vi "Initialize.vi"(8 "error in (no error)":errorcluster, 11 "Serial Config":T1={"Baud"=9600, "Flow Ctl"=0, "Parity"=0, "COM Port"="", "Address"=0} {"Parity" items=["None", "Odd", "Even"]; "Flow Ctl" items=["None"]; "Baud" items=["4800"=4800, "9600"=9600, "19200"=19200, "38400"=38400]}) -> (0 "error out":errorcluster, 3 "Serial Config 2":T1={"Baud"=9600, "Flow Ctl"=0, "Parity"=0, "COM Port"="", "Address"=0} {"Parity" items=["None", "Odd", "Even"]; "Flow Ctl" items=["None"]; "Baud" items=["4800"=4800, "9600"=9600, "19200"=19200, "38400"=38400]})   [LabVIEW 2014, in "Omega CN9600 series.lvclass"]
uses:
  Omega CN9600 series.lvclass
  Serial_Config_Omega.ctl
  <vilib>/Instr/_visa.llb/VISA Set IO Buffer Mask.ctl
  <vilib>/Utility/error.llb/Error Cluster From Error Code.vi
  <vilib>/ErrorRing/Error Ring.xnode
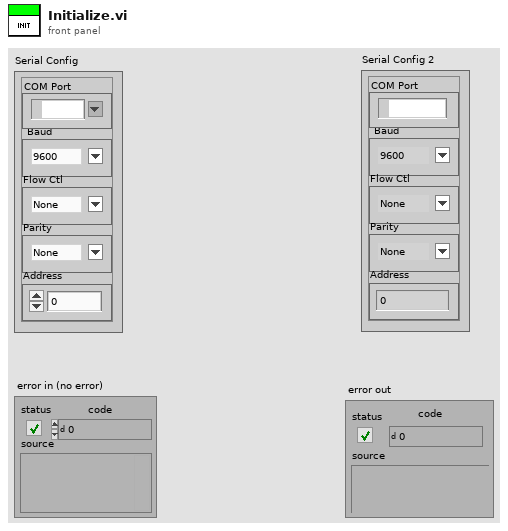
[diagram p1: front panel]
types:
  T1 = typedef "Omega CN9600 series.lvclass/Serial_Config_Omega.ctl" = cluster{"Baud":u32, "Flow Ctl":u16, "Parity":u16, "COM Port":refnum<visa-resource-name>, "Address":u8}
  T2 = typedef "VISA Set IO Buffer Mask.ctl" = u16
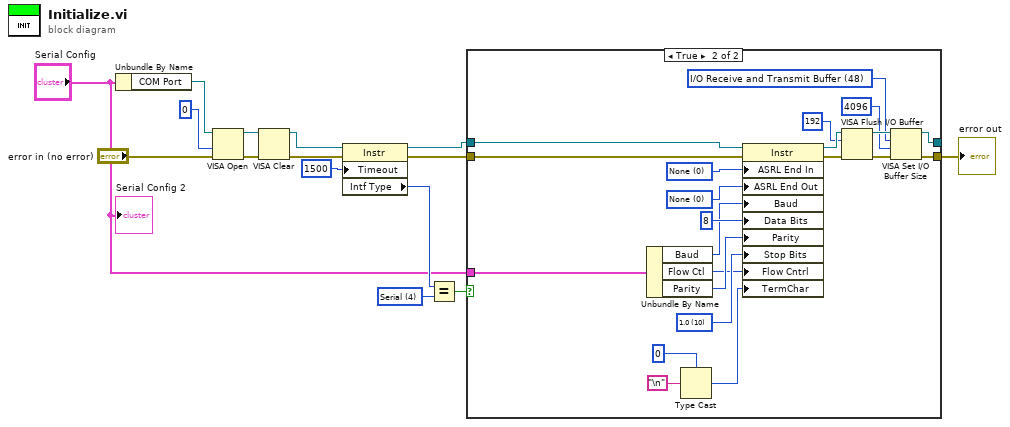
[diagram p0: block diagram]
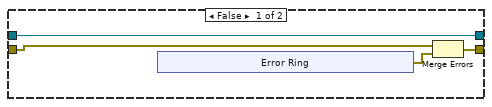
[diagram p2: hidden frame]
diagram:
  w7 = u16 4 items=["GPIB"=1, "VXI"=2, "GPIB-VXI"=3, "Serial"=4, "PXI"=5, "TCPIP"=6, "USB"=7] ("Interface Information:Interface Type")
  n1 = Unbundle By Name("Serial Config") -> ("COM Port"=w3:refnum<visa-resource-name>)
  n2 = VISA Open(access mode=0, error in (no error)="error in (no error)", VISA resource name=w3) -> (VISA resource name=w12:refnum<visa-resource-name>, error out=w13:errorcluster)  [unwired: 2 in]
  n3 = VISA Clear(VISA resource name=w12, error in (no error)=w13) -> (VISA resource name out=w11:refnum<visa-resource-name>, error out=w10:errorcluster)
  n4 = property class="Instr"(reference=w11, error in=w10, "Timeout"=u32 1500 ("General Settings:Timeout Value")) -> (reference out=w5:refnum<visa-resource-name>, error out=w4:errorcluster, "Intf Type"=w8:u16)
  n5 = Equal?(x=w8, y=w7) -> (x = y?=w6:bool)
  n6 = case shown="True" w6 {
    tunnel: w5 -> [w19 w45]
    tunnel: w4 -> [w16 w44]
    tunnel: [w19 w27] -> _
    tunnel: [w17 w26] -> w2
    tunnel: "Serial Config" -> [_ w25]
    frame False {
      n7 = xnode "Error Ring"() -> ("error out"=w18:errorcluster)
      n8 = Merge Errors(w16, w18) -> (w17:errorcluster)
    }
    frame True {
      w24 = u16 0 items=["None", "Last Bit", "TermChar", "Break"] ("Serial Settings:End Mode for Writes")
      w29 = T2 48 items=["I/O Receive Buffer"=16, "I/O Transmit Buffer"=32, "I/O Receive and Transmit Buffer"=48] ("Mask")
      w35 = u16 0 items=["None", "Last Bit", "TermChar", "Break"] ("Serial Settings:End Mode for Writes")
      w41 = u16 10 items=["1.0"=10, "1.5"=15, "2.0"=20] ("Serial Settings:Stop Bits")
      n9 = Unbundle By Name(w25) -> ("Baud"=w36:u32, "Flow Ctl"=w40:u16, "Parity"=w42:u16)
      n10 = Type Cast(type=u8 0, x="\n") -> (*(type *) &x=w37:u8)
      n11 = property class="Instr"(reference=w45, error in=w44, "ASRL End In"=w35, "ASRL End Out"=w24, "Baud"=w36, "Data Bits"=u16 8 ("Serial Settings:Data Bits"), "Parity"=w42, "Stop Bits"=w41, "Flow Cntrl"=w40, "TermChar"=w37) -> (reference out=w34:refnum<visa-resource-name>, error out=w33:errorcluster)
      n12 = VISA Flush I/O Buffer(VISA resource name=w34, mask (16)=192, error in (no error)=w33) -> (VISA resource name out=w31:refnum<visa-resource-name>, error out=w30:errorcluster)
      n13 = VISA Set I/O Buffer Size(VISA resource name=w31, mask (16)=w29, size (4096)=u32 4096, error in (no error)=w30) -> (VISA resource name out=w27:refnum<visa-resource-name>, error out=w26:errorcluster)
    }
  }
  "error out" <- w2
  "Serial Config 2" <- "Serial Config"
